vi "FPGAmain_5782_AM_PID_v2.vi"() -> ()   [LabVIEW 2013]
uses:
  FPGA/DataMode.ctl
  FPGA/Input_5782/5782_states.ctl
  <vilib>/Platform/TimedLoop/XDataNode/timing_clust.ctl
  <vilib>/Platform/TimedLoop/XDataNode/nitl_modes.ctl
  <vilib>/Platform/TimedLoop/XDataNode/wakeup.ctl
  <vilib>/rvi/Emulation/niFpgaSctlEmulationGetInTimedLoop.vi
  <vilib>/rvi/Emulation/niFpgaEmulationReportErrorSimple.vi
  <vilib>/rvi/Emulation/niFpgaGetClockAttributes.vi
  <vilib>/rvi/eio/common/nirviEmuTemplateMethod_errors.vi
  <vilib>/rvi/Emulation/niFpgaCriticalErrorInLSC.vi
  <vilib>/rvi/DataTransferAndStorage/Register/Emulation/niFpgaRegisterEmulationFpgaImpl.vi
  <instcachedir>/0/niFpgaRegisterEmulationFpgaImpl_DCF4BC0110594B98B44A971D60CEEC4D.lvgen/niFpgaRegisterEmulationFpgaImpl_DCF4BC0110594B98B44A971D60CEEC4D_005.vi
  <vilib>/rvi/DataTransferAndStorage/Container/Common/niFpgaContainerGetUniqueNameForEmu.vi
  <instcachedir>/0/niFpgaRegisterEmulationFpgaImpl_DCF4BC0110594B98B44A971D60CEEC4D.lvgen/niFpgaRegisterEmulationFpgaImpl_DCF4BC0110594B98B44A971D60CEEC4D_016.vi
  <instcachedir>/0/niFpgaRegisterEmulationFpgaImpl_DCF4BC0110594B98B44A971D60CEEC4D.lvgen/niFpgaRegisterEmulationFpgaImpl_DCF4BC0110594B98B44A971D60CEEC4D_017.vi
  <instcachedir>/0/niFpgaRegisterEmulationFpgaImpl_DCF4BC0110594B98B44A971D60CEEC4D.lvgen/niFpgaRegisterEmulationFpgaImpl_DCF4BC0110594B98B44A971D60CEEC4D_012.vi
  <instcachedir>/0/niFpgaRegisterEmulationFpgaImpl_DCF4BC0110594B98B44A971D60CEEC4D.lvgen/niFpgaRegisterEmulationFpgaImpl_DCF4BC0110594B98B44A971D60CEEC4D_015.vi
  <vilib>/rvi/FIFO/Fifo_Resource/nirvififoEmulationReadFpgaImpl.vi
  <vilib>/rvi/interface/RandomDataEmulation/nirviRandomDataMultiElementFPGAFIFO.vi
  <instcachedir>/0/nirviRandomDataMultiElementFPGAFIFO_F2B80EDE0D7944A08478D8D26097D4DB.lvgen/nirviRandomDataMultiElementFPGAFIFO_F2B80EDE0D7944A08478D8D26097D4DB_005.vi
  <vilib>/rvi/interface/RandomDataEmulation/niFpgaRandomDataHandleErrors.vi
  <instcachedir>/0/niFpgaRegisterEmulationFpgaImpl_DCF4BC0110594B98B44A971D60CEEC4D.lvgen/niFpgaRegisterEmulationFpgaImpl_DCF4BC0110594B98B44A971D60CEEC4D_009.vi
  <vilib>/rvi/interface/RandomDataEmulation/nirviRandomDataFPGAFIFO.vi
  <vilib>/rvi/FIFO/Fifo_Resource/nirvififoEmulationWriteFpgaImpl.vi
  <vilib>/Platform/TimedLoop/XDataNode/XDataNode.xnode
  <vilib>/eio/EIONode/EIONode.xnode
  <vilib>/rvi/DataTransferAndStorage/Container/XNode/niFpgaContainer.xnode
  <vilib>/rvi/DataTransferAndStorage/Register/Emulation/niFpgaRegisterEmulation.vi
  <vilib>/rvi/FIFO/Fifo_Resource/nirvififoEmulationRead.vi
  <vilib>/rvi/interface/RandomDataEmulation/nirviRandomDataFpgaMultiElementTemplate.vi
  <vilib>/rvi/interface/RandomDataEmulation/nirviRandomDataFpgaReadWriteTemplate.vi
  <vilib>/rvi/FIFO/Fifo_Resource/nirvififoEmulationWrite.vi
  <vilib>/Platform/TimedLoop/XDataNode/XDNodeRunTimeDep.lvlib
panel:
  in  "IO Module\\AO Data Sync":bool=TRUE
  in  "IO Module\\SPI Write Data":u16
  out "IO Module\\SPI Read Data":u8
  in  "IO Module\\SPI Read":bool
  in  "IO Module\\SPI Write":bool
  in  "IO Module\\SPI Address":u16
  in  "IO Module\\SPI Device":u8
  out "IO Module\\SPI Idle":bool
  in  "AM phase":fxp<+,64,64>
  in  "delay phase":fxp<+,64,64>
  in  "User Command Commit":bool
  in  "User Command":u8
  out "User Command Idle":bool
  out "User Command Status":u8
  in  "User Data 0":u8
  in  "User Data 1":u8
  out "PLL Locked":bool
  out "User Error":bool
  out "Configured?":bool
  in  "Continuous":bool
  in  "5782 record length":u16=4000 caption="Samples Per Trigger" min=1 step=1
  in  "Trigger Acquisition":bool
  out "IO Module\\Trigger Input":bool
  in  "Downsample":fxp<+,8,8>=1.0
  in  "new coeffs":bool
  in  "FIR coeffs":fxp<+/-,18,18>[](array[numeric])
  in  "CIC Gain":fxp<+/-,32,1>=0.00390625 format="%#_32g"
  in  "Acquisition running":bool
  in  "Phase output":fxp<+,64,64>[](array[numeric])=[0.0, 0.0, 0.0, 0.0, 0.0, 0.0, 0.0, 0.0]
  in  "Simulated phase 5782":fxp<+,64,64>[](array[numeric])=[0.0, 0.0]
  in  "Mode":T1
  in  "Phase 5782":fxp<+,64,64>[](array[numeric])=[0.0, 0.0]
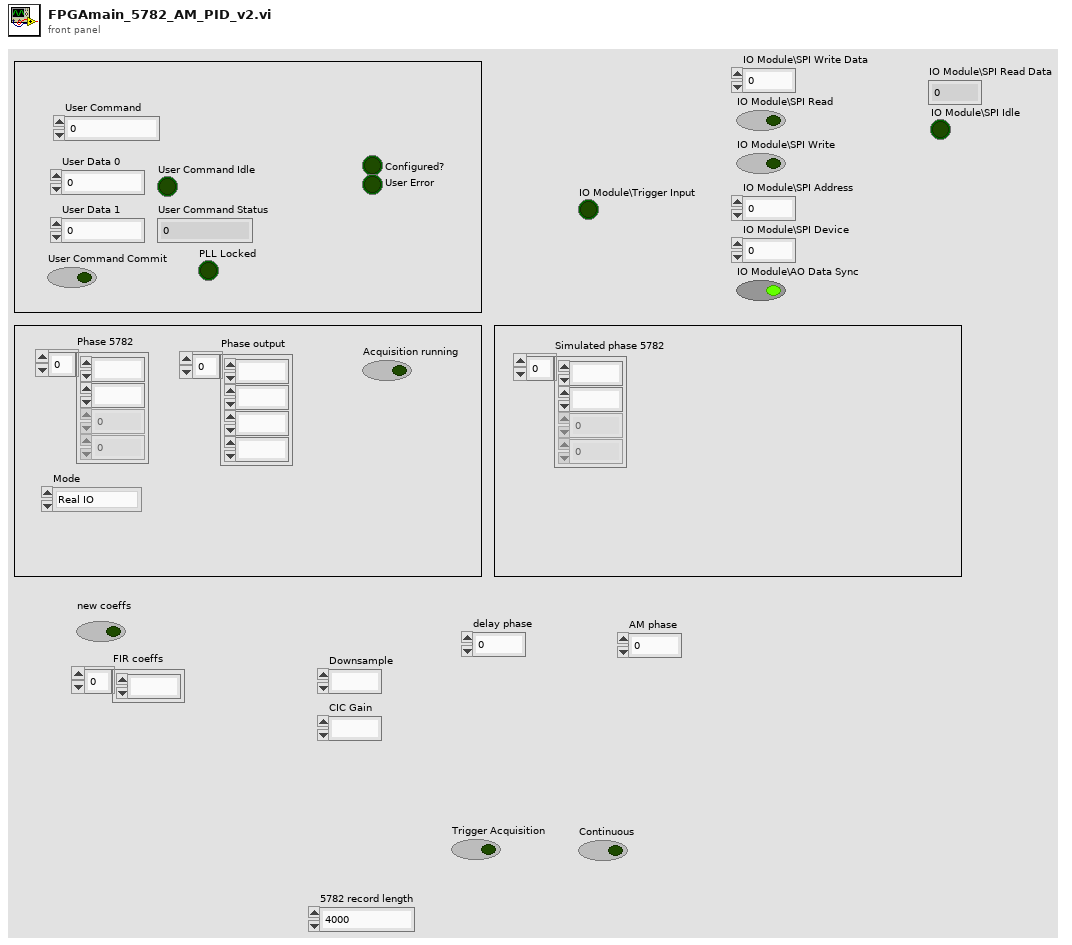
[diagram p1: front panel]
types:
  T1 = typedef "DataMode.ctl" = enum16{"Real IO", "Simulated"}
  T2 = typedef "5782_states.ctl" = enum8{"Wait for trigger", "Acquisition", "Send record length", "Quiet period"}
  T3 = typedef "XDNodeRunTimeDep.lvlib/timing_clust.ctl" = cluster{"Expected End [f-1]":u64, "Actual End [f-1]":u64, "Finished Late? [f-1]":bool, "Expected End [i-1]":u64, "Actual End [i-1]":u64, "Finished Late? [i-1]":bool, "Expected Start [i]":u64, "Actual Start [i]":u64, "Expected Start [f]":u64, "Actual Start [f]":u64, "Source Name":string, "Structure Name":string, "Period":i64, "Deadline":i64, "Offset":i64, "Start":i64, "Priority":i32, "Timeout":i32, "Mode":T4, "Wakeup Reason":T5, "Error":errorcluster, "Source Type":string, "Secondary Source Type":string, "Global End Time":u64, "Global Start Time":u64, "Frame Duration":u64, "Iteration Duration":u64, "Assigned CPU":i32, "I/O Scan Engine Mode":u32}
  T4 = typedef "XDNodeRunTimeDep.lvlib/nitl_modes.ctl" = enum32{"No Change", "Process missed periods, maintain original phase", "Discard missed periods, maintain original phase", "Process missed periods, ignore original phase", "Discard missed periods, ignore original phase"}
  T5 = typedef "XDNodeRunTimeDep.lvlib/wakeup.ctl" = enum32{"Normal", "Aborted", "Asynchronous wakeup", "Timing source error", "Timed loop error", "Timeout"}
  T6 = typedef "I16 array size 2.ctl" = i16[]
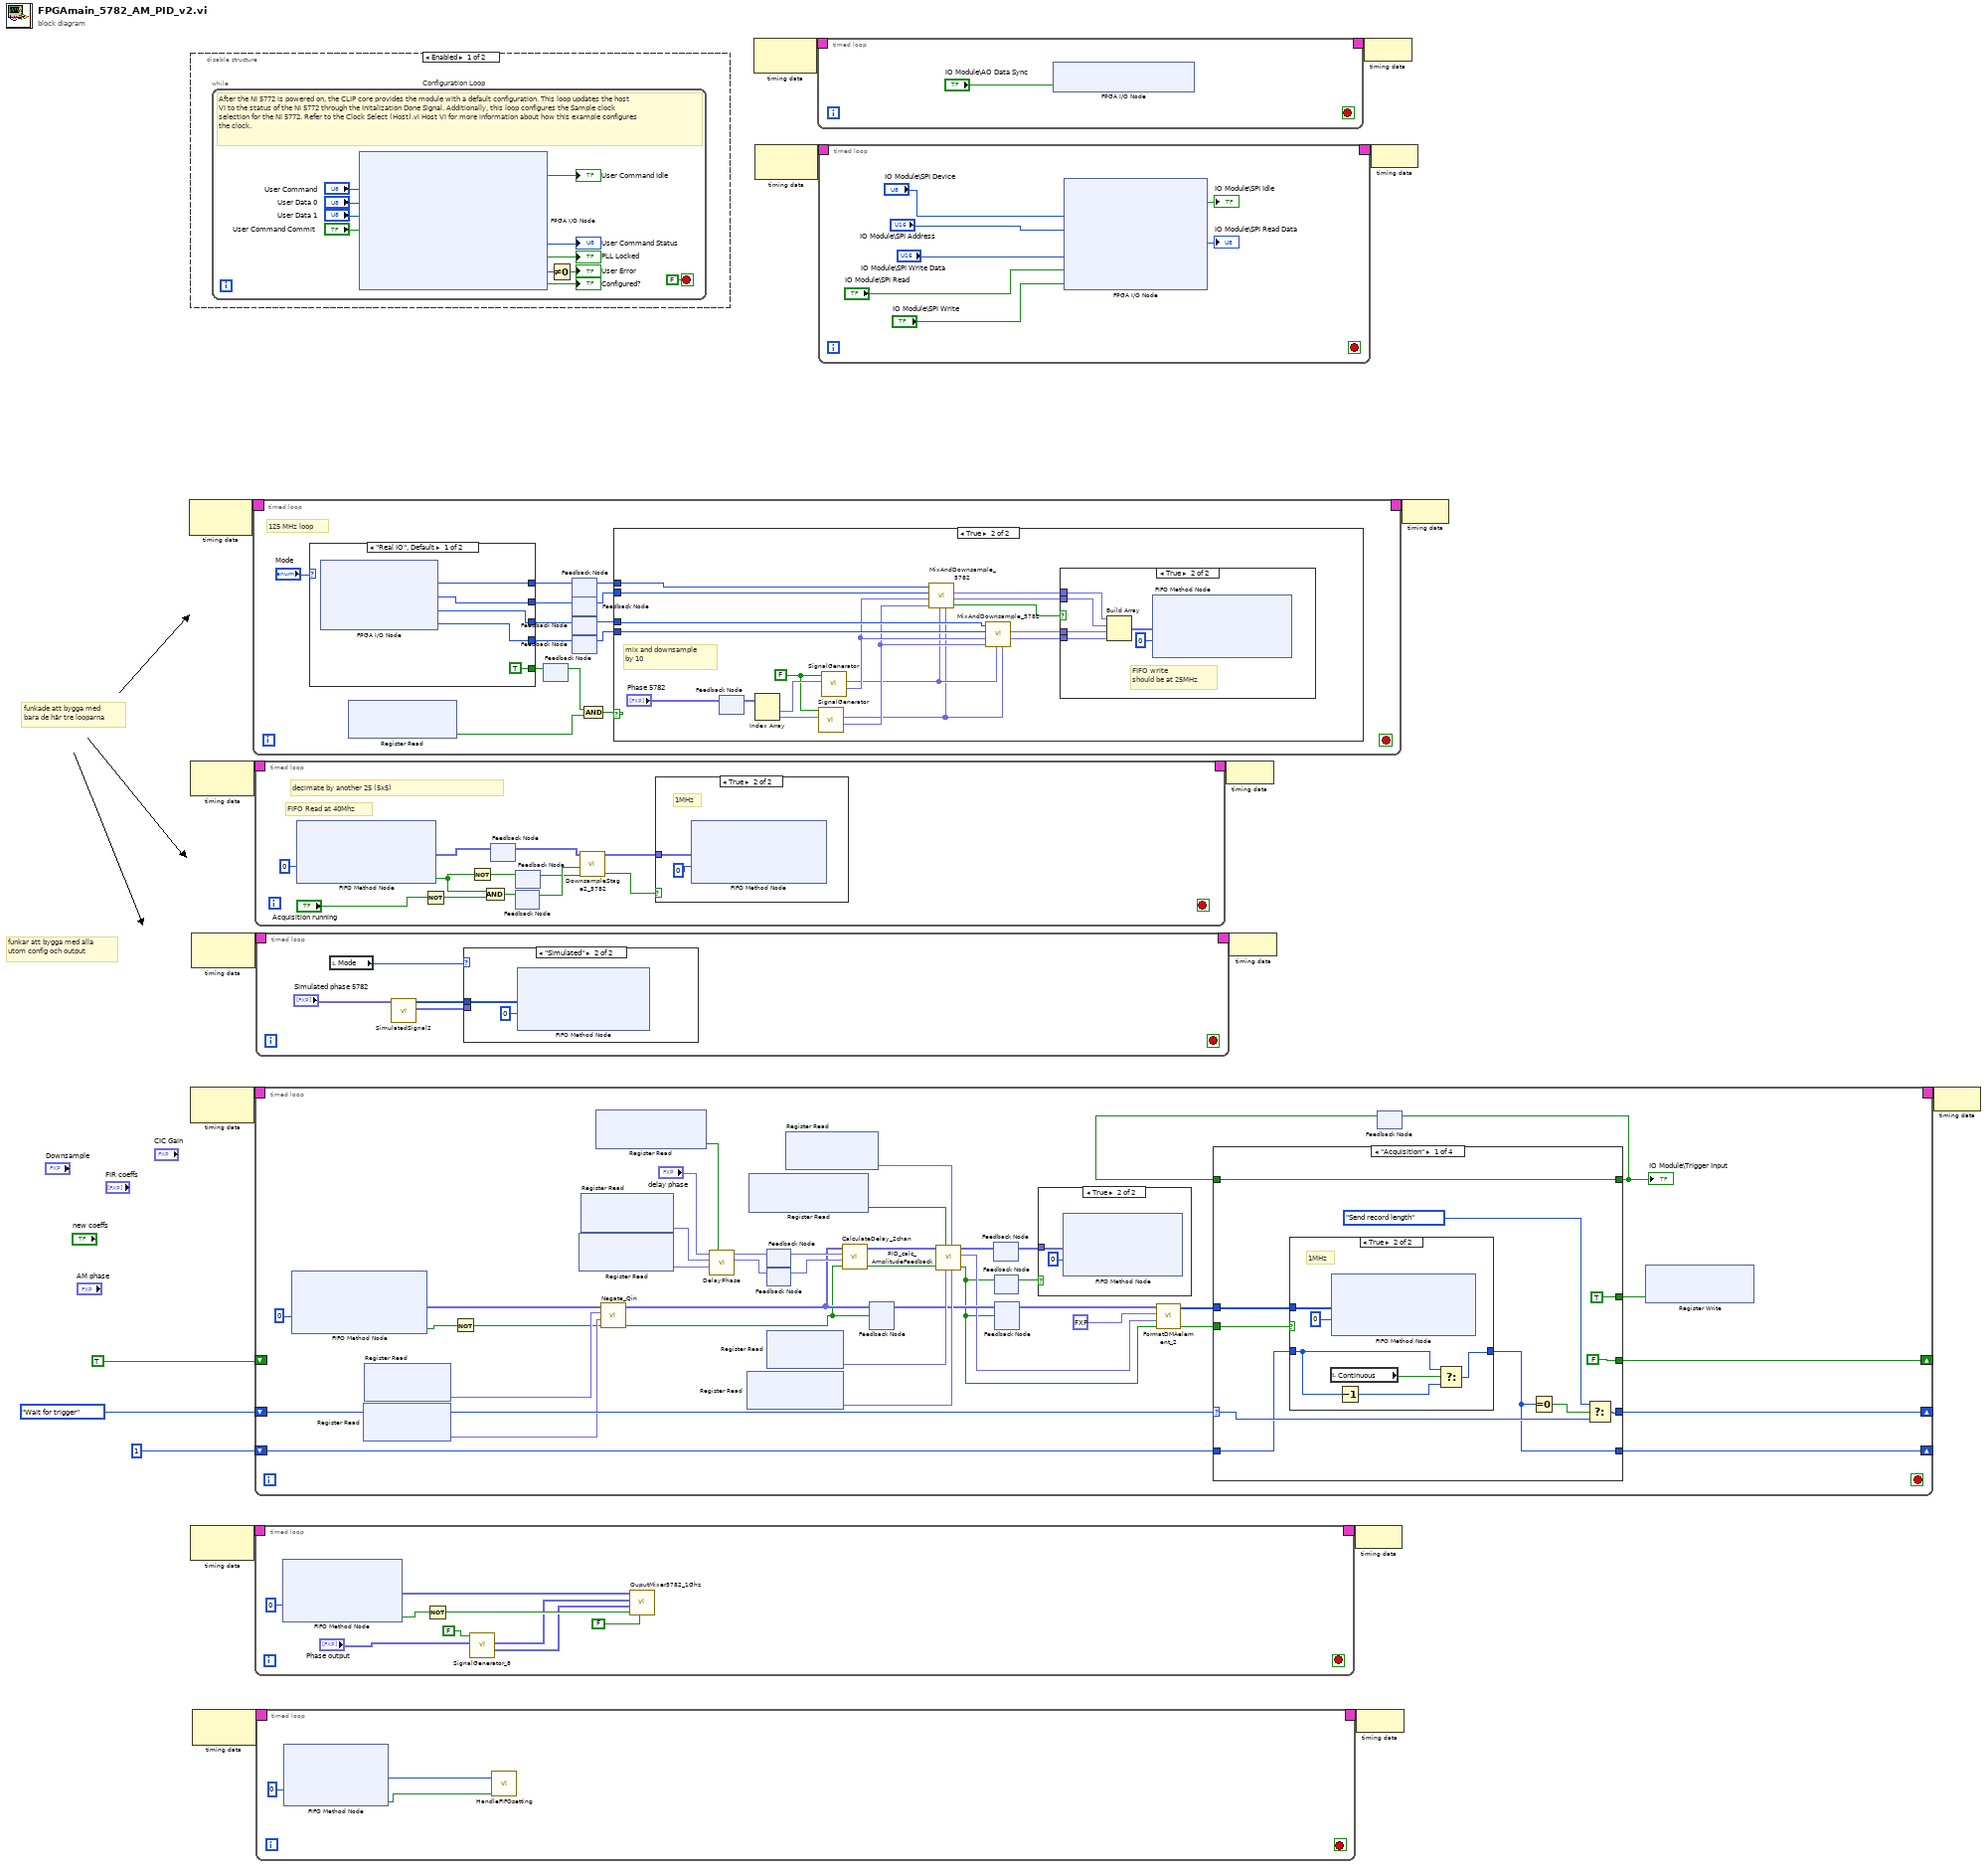
[diagram p0: block diagram]
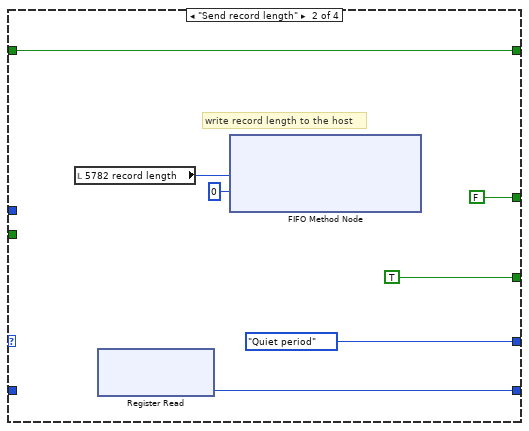
[diagram p4: hidden frame]
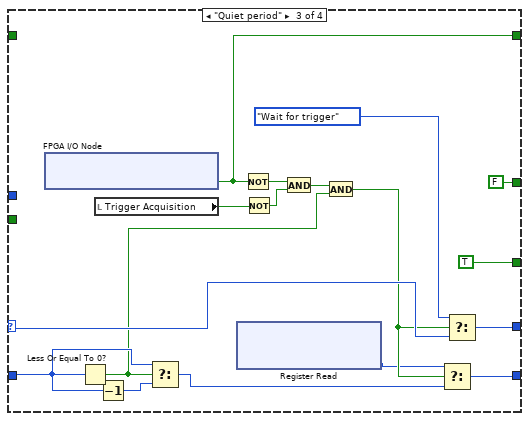
[diagram p5: hidden frame]
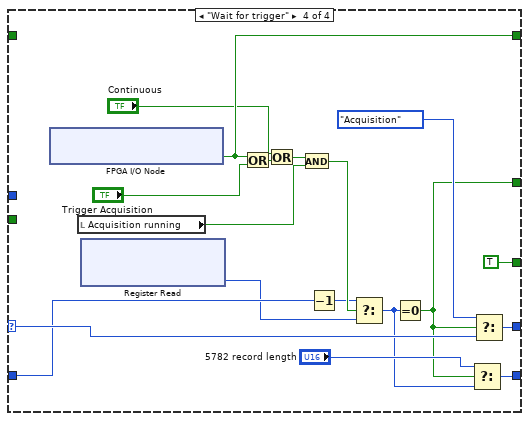
[diagram p6: hidden frame]
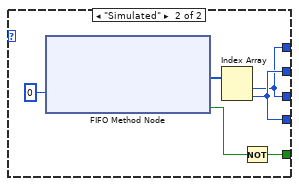
[diagram p10: hidden frame]
diagram:
  # "funkar att bygga med alla\nutom config och output"
  # "funkade att bygga med\nbara de här tre looparna"
  n1 = node-c288() -> (w15:T3)  [unwired: 1 in]
  n2 = disable-structure shown="Enabled" {
    frame Enabled {
      n3 = while "Configuration Loop" {
        stop <- FALSE stop-if-true
        # "After the NI 5772 is powered on, the CLIP core provides the module with a default configuration. This loop updates the host VI to the status of the NI 5772 through the Initalization Done Signal. Additionally, this loop configures the Sample clock selection for the NI 5772. Refer to the Clock Select (Host).vi Host VI for more information about how this example configures the clock."
        n4 = xnode "FPGA I/O Node"("IO Module\\User Command"="User Command", "IO Module\\User Data 0"="User Data 0", "IO Module\\User Data 1"="User Data 1", "IO Module\\User Command Commit"="User Command Commit") -> ("IO Module\\User Command Idle"=→"User Command Idle":bool, "IO Module\\User Command Status"=→"User Command Status":u8, "IO Module\\PLL Locked"=→"PLL Locked":bool, "IO Module\\User Error"=w25:u8, "IO Module\\Initialization Done"=→"Configured?":bool)  [unwired: 9 in, 9 out]
        n5 = Not Equal To 0?(x=w25) -> (x != 0?=→"User Error":bool)
      }
    }
    frame Disabled {
    }
  }
  n6 = node-c288() -> (w19:T3)  [unwired: 1 in]
  n7 = node-c288() -> (w13:T3)  [unwired: 1 in]
  n8 = node-c288() -> (w6:T3)  [unwired: 1 in]
  n9 = node-c288() -> (w17:T3)  [unwired: 1 in]
  n10 = node-c288() -> (w8:T3)  [unwired: 1 in]
  n11 = timed-loop {
    timing: w15 -> [_]
    timing-out: [_] -> w14
    stop <- _ stop-if-true
    # "125 MHz loop"
    n12 = case shown="\"Real IO\", Default" "Mode" {
      tunnel: [w72 w75] -> w41
      tunnel: [w71 w76] -> w39
      tunnel: [w70 w75] -> w37
      tunnel: [w69 w76] -> w34
      tunnel: [TRUE w73] -> w33
      frame "Real IO", Default {
        n13 = xnode "FPGA I/O Node"() -> ("IO Module\\AI 0 N-1"=w72:i16, "IO Module\\AI 0 N"=w71:i16, "IO Module\\AI 1 N-1"=w70:i16, "IO Module\\AI 1 N"=w69:i16)  [unwired: 4 in, 4 out]
      }
      frame "Simulated" {
        n14 = xnode ("FIFO Method Node")("Timeout"=0) -> ("Element"=w77:i16[], "Timed Out?"=w74:bool)  [unwired: 1 in, 1 out]
        n15 = Index Array(array=w77) -> (element #1=w75:i16, element #2=w76:i16)  [unwired: 2 in]
        n16 = Not(x=w74) -> (.not. x?=w73:bool)
      }
    }
    n17 = xnode ("Register Read")() -> ("Data"=w31:bool)  [unwired: 1 in, 1 out]
    n18 = feedback #1() -> (w32:bool)  [unwired: 1 in]
    n19 = feedback-in #1(w33) -> ()
    n20 = feedback #2() -> (w40:i16)  [unwired: 1 in]
    n21 = feedback-in #2(w41) -> ()
    n22 = feedback #3() -> (w38:i16)  [unwired: 1 in]
    n23 = feedback-in #3(w39) -> ()
    n24 = feedback #4() -> (w36:i16)  [unwired: 1 in]
    n25 = feedback-in #4(w37) -> ()
    n26 = feedback #5() -> (w35:i16)  [unwired: 1 in]
    n27 = feedback-in #5(w34) -> ()
    n28 = And(x=w32, y=w31) -> (x .and. y?=w42:bool)
    n29 = case shown="True" w42 {
      tunnel: w40 -> [_ w51]
      tunnel: w38 -> [_ w50]
      tunnel: w36 -> [_ w49]
      tunnel: w35 -> [_ w48]
      frame False {
      }
      frame True {
        w52 = FALSE
        # "mix and downsample\nby 10"
        n30 = feedback #6() -> (w55:fxp<+,64,64>[])  [unwired: 1 in]
        n31 = feedback-in #6("Phase 5782") -> ()
        n32 = Index Array(array=w55) -> (element #1=w54:fxp<+,64,64>, element #2=w56:fxp<+,64,64>)  [unwired: 2 in]
        n33 = call "SignalGenerator.vi"("phase"=w56, "Reset"=w52) -> ("Cos"=w46:fxp<+/-,16,0>, "Sin"=w44:fxp<+/-,16,0>)  [unwired: 7 in, 1 out]
        n34 = call "SignalGenerator.vi"("phase"=w54, "Reset"=w52) -> ("Cos"=w47:fxp<+/-,16,0>, "Sin"=w45:fxp<+/-,16,0>)  [unwired: 7 in, 1 out]
        n35 = call "MixAndDownsample_5782.vi"("sin1"=w44, "sin0"=w45, "cos1"=w46, "cos0"=w47, "signal 1"=w50, "signal 0"=w51) -> ("data valid"=w59:bool, "Q out"=w60:fxp<+/-,16,14>, "I out"=w61:fxp<+/-,16,14>)  [unwired: 3 in]
        n36 = call "MixAndDownsample_5782.vi"("sin1"=w44, "sin0"=w45, "cos1"=w46, "cos0"=w47, "signal 1"=w48, "signal 0"=w49) -> ("Q out"=w57:fxp<+/-,16,14>, "I out"=w58:fxp<+/-,16,14>)  [unwired: 3 in, 1 out]
        n37 = case shown="True" w59 {
          tunnel: w60 -> [_ w67]
          tunnel: w61 -> [_ w64]
          tunnel: w58 -> [_ w63]
          tunnel: w57 -> [_ w62]
          frame False {
          }
          frame True {
            # "FIFO write\nshould be at 25MHz"
            n38 = Build Array(w64, w67, w63, w62) -> (w66:fxp<+/-,16,14>[])
            n39 = xnode ("FIFO Method Node")("Element"=w66, "Timeout"=0) -> ()  [unwired: 1 in, 2 out]
          }
        }
      }
    }
  }
  n40 = timed-loop {
    timing: w19 -> [_]
    timing-out: [_] -> w18
    stop <- _ stop-if-true
    # "FIFO Read at 40Mhz"
    # "decimate by another 25 (5x5)"
    n41 = xnode ("FIFO Method Node")("Timeout"=0) -> ("Element"=w86:fxp<+/-,16,14>[], "Timed Out?"=w88:bool)  [unwired: 1 in, 1 out]
    n42 = Not(x="Acquisition running") -> (.not. x?=w89:bool)
    n43 = Not(x=w88) -> (.not. x?=w82:bool)
    n44 = And(x=w88, y=w89) -> (x .and. y?=w84:bool)
    n45 = feedback #7() -> (w85:fxp<+/-,16,14>[])  [unwired: 1 in]
    n46 = feedback-in #7(w86) -> ()
    n47 = feedback #8() -> (w83:bool)  [unwired: 1 in]
    n48 = feedback-in #8(w84) -> ()
    n49 = feedback #9() -> (w81:bool)  [unwired: 1 in]
    n50 = feedback-in #9(w82) -> ()
    n51 = call "DownsampleStage2_5782.vi"("valid in"=w81, "reset"=w83, "Data in"=w85) -> ("valid out"=w90:bool, "data out"=w91:fxp<+/-,16,14>[])  [unwired: 7 in]
    n52 = case shown="True" w90 {
      tunnel: w91 -> [_ w93]
      frame False {
      }
      frame True {
        # "1MHz"
        n53 = xnode ("FIFO Method Node")("Element"=w93, "Timeout"=0) -> ()  [unwired: 1 in, 2 out]
      }
    }
  }
  n54 = timed-loop {
    timing: w13 -> [_]
    timing-out: [_] -> w12
    shift-right: [w134] -> _
    shift-left: 5782_states."Wait for trigger" ("5782 states") -> [w136]
    shift-right: [w133] -> _
    shift-left: u16 1 ("trigger samples") -> [w135]
    shift-right: [w128] -> _
    shift-left: TRUE -> [_]
    stop <- _ stop-if-true
    n55 = xnode ("FIFO Method Node")("Timeout"=0) -> ("Element"=w107:fxp<+/-,16,14>[], "Timed Out?"=w131:bool)  [unwired: 1 in, 1 out]
    n56 = xnode ("Register Read")() -> ("Data"=w118:fxp<+/-,16,14>)  [unwired: 1 in, 1 out]
    n57 = xnode ("Register Read")() -> ("Data"=w119:fxp<+/-,16,14>)  [unwired: 1 in, 1 out]
    n58 = Not(x=w131) -> (.not. x?=w108:bool)
    n59 = xnode ("Register Read")() -> ("Data"=w115:fxp<+/-,16,0>)  [unwired: 1 in, 1 out]
    n60 = xnode ("Register Read")() -> ("Data"=w116:fxp<+/-,16,0>)  [unwired: 1 in, 1 out]
    n61 = xnode ("Register Read")() -> ("Data"=w117:bool)  [unwired: 1 in, 1 out]
    n62 = call "Negate_Qin.vi"("valid in"=w108, "DC offset chan 1"=w118, "DC offset chan 0"=w119, "Data in"=w107) -> ("valid out"=w101:bool, "Data out"=w102:fxp<+/-,16,14>[])  [unwired: 6 in]
    n63 = call "DelayPhase.vi"("Use fixed delay"=w117, "fixed cos_fi"=w115, "fixed sin fi"=w116, "delay phase"="delay phase") -> ("cos_fi"=w120:fxp<+/-,16,0>, "sin fi"=w121:fxp<+/-,16,0>)  [unwired: 6 in]
    n64 = xnode ("Register Read")() -> ("Data"=w110:fxp<+/-,32,6>)  [unwired: 1 in, 1 out]
    n65 = xnode ("Register Read")() -> ("Data"=w112:bool)  [unwired: 1 in, 1 out]
    n66 = feedback-in #10(w121) -> ()
    n67 = feedback #10() -> (w124:fxp<+/-,16,0>)  [unwired: 1 in]
    n68 = feedback #11() -> (w123:fxp<+/-,16,0>)  [unwired: 1 in]
    n69 = feedback-in #11(w120) -> ()
    n70 = xnode ("Register Read")() -> ("Data"=w111:fxp<+/-,32,6>)  [unwired: 1 in, 1 out]
    n71 = xnode ("Register Read")() -> ("Data"=w109:fxp<+/-,32,6>)  [unwired: 1 in, 1 out]
    n72 = call "CalculateDelay_2chan.vi"("input valid"=w101, "cos_fi"=w123, "sin fi"=w124, "Data in"=w102) -> ("output valid"=w113:bool, "Data out"=w114:fxp<+/-,16,14>[])  [unwired: 6 in]
    n73 = feedback #12() -> (w103:fxp<+/-,16,14>[])  [unwired: 1 in]
    n74 = feedback-in #12(w102, w101) -> ()
    n75 = call "PID_calc_AmplitudeFeedback.vi"("Kd/Tau"=w110, "Ki*Tau"=w109, "Kp"=w111, "Enabled"=w112, "input valid"=w113, "Data in"=w114) -> ("output valid"=w97:bool, "c(t)"=w99:fxp<+/-,32,21>, "data out"=w106:fxp<+/-,16,14>[])  [unwired: 2 in, 1 out]
    n76 = feedback #13() -> (w105:fxp<+/-,16,14>[])  [unwired: 1 in]
    n77 = feedback-in #13(w106) -> ()
    n78 = feedback #14() -> (w104:bool)  [unwired: 1 in]
    n79 = feedback-in #14(w97) -> ()
    n80 = feedback #15() -> (w100:fxp<+/-,16,14>[])  [unwired: 1 in]
    n81 = feedback-in #15(w103, w97) -> ()
    n82 = case shown="True" w104 {
      tunnel: w105 -> [_ w137]
      frame False {
      }
      frame True {
        n83 = xnode ("FIFO Method Node")("Element"=w137, "Timeout"=0) -> ()  [unwired: 1 in, 2 out]
      }
    }
    n84 = call "FormatDMAelement_2.vi"("valid in"=w97, "c(t) - AM"=w99, "c(t) - Phase"=fxp<+/-,32,21> 0.0, "Data in"=w100) -> ("valid out"=w129:bool, "Element"=w130:u64[])  [unwired: 6 in]
    n85 = feedback #16() -> (w126:bool)  [unwired: 1 in]
    n86 = case shown="\"Acquisition\"" w136 {
      selector: w136 -> [w149 _ w179 w198]
      tunnel: w135 -> [w145 _ w167 w185]
      tunnel: [w148 5782_states."Quiet period" ("5782 states") w178 w197] -> w134
      tunnel: [w142 w157 w180 w196] -> w133
      tunnel: w130 -> [w143 _ _ _]
      tunnel: w129 -> [w144 _ _ _]
      tunnel: [FALSE TRUE TRUE TRUE] -> w128
      tunnel: [TRUE FALSE ("5782 triggered") FALSE ("5782 triggered") w189] -> w127
      tunnel: [w141 w158 w169 w188] -> w125
      tunnel: w126 -> [w141 w158 _ _]
      frame "Acquisition" {
        n87 = case shown="True" w144 {
          tunnel: w143 -> [_ w156]
          tunnel: [w150 w153] -> w142
          tunnel: w145 -> [w150 w151]
          frame False {
          }
          frame True {
            # "1MHz"
            n88 = local read "Continuous"() -> (w154:bool)
            n89 = xnode ("FIFO Method Node")("Element"=w156, "Timeout"=0) -> ()  [unwired: 1 in, 2 out]
            n90 = Decrement(x=w151) -> (x-1=w152:u16)
            n91 = Select(t=w151, s=w154, f=w152) -> (s? t:f=w153:u16)
          }
        }
        n92 = Equal To 0?(x=w142) -> (x = 0?=w146:bool)
        n93 = Select(t=5782_states."Send record length" ("5782 states"), s=w146, f=w149) -> (s? t:f=w148:T2)
      }
      frame "Send record length" {
        # "write record length to the host"
        n94 = local read "5782 record length"() -> (w160:u16)
        n95 = xnode ("Register Read")() -> ("Data"=w157:u16)  [unwired: 1 in, 1 out]
        n96 = xnode ("FIFO Method Node")("Element"=w160, "Timeout"=0) -> ()  [unwired: 1 in, 2 out]
      }
      frame "Quiet period" {
        n97 = xnode "FPGA I/O Node"() -> ("IO Module\\Trigger Input"=w169:bool)  [unwired: 1 in, 1 out]
        n98 = Less Or Equal To 0?(x=w167) -> (x <= 0?=w166:bool)
        n99 = local read "Trigger Acquisition"() -> (w175:bool)
        n100 = Decrement(x=w167) -> (x-1=w168:u16)
        n101 = Select(t=w167, s=w166, f=w168) -> (s? t:f=w165:u16)
        n102 = xnode ("Register Read")() -> ("Data"=w164:u16)  [unwired: 1 in, 1 out]
        n103 = Not(x=w169) -> (.not. x?=w174:bool)
        n104 = Not(x=w175) -> (.not. x?=w173:bool)
        n105 = And(x=w174, y=w173) -> (x .and. y?=w172:bool)
        n106 = And(x=w172, y=w166) -> (x .and. y?=w177:bool)
        n107 = Select(t=w164, s=w177, f=w165) -> (s? t:f=w180:u16)
        n108 = Select(t=5782_states."Wait for trigger" ("5782 states"), s=w177, f=w179) -> (s? t:f=w178:T2)
      }
      frame "Wait for trigger" {
        n109 = xnode "FPGA I/O Node"() -> ("IO Module\\Trigger Input"=w188:bool)  [unwired: 1 in, 1 out]
        n110 = local read "Acquisition running"() -> (w190:bool)
        n111 = xnode ("Register Read")() -> ("Data"=w181:u16)  [unwired: 1 in, 1 out]
        n112 = Or(x=w188, y="Trigger Acquisition") -> (x .or. y?=w184:bool)
        n113 = Or(x="Continuous", y=w184) -> (x .or. y?=w182:bool)
        n114 = And(x=w182, y=w190) -> (x .and. y?=w191:bool)
        n115 = Decrement(x=w185) -> (x-1=w186:u16)
        n116 = Select(t=w186, s=w191, f=w181) -> (s? t:f=w187:u16)
        n117 = Equal To 0?(x=w187) -> (x = 0?=w189:bool)
        n118 = Select(t="5782 record length", s=w189, f=w187) -> (s? t:f=w196:u16)
        n119 = Select(t=5782_states."Acquisition" ("5782 states"), s=w189, f=w198) -> (s? t:f=w197:T2)
      }
    }
    "IO Module\\Trigger Input" <- w125
    n120 = feedback-in #16(w125) -> ()
    n121 = xnode ("Register Write")("Data"=w127) -> ()  [unwired: 1 in, 1 out]
  }
  n122 = timed-loop {
    timing: w6 -> [_]
    timing-out: [_] -> w5
    stop <- _ stop-if-true
    n123 = xnode ("FIFO Method Node")("Timeout"=0) -> ("Element"=w205:fxp<+/-,16,14>[], "Timed Out?"=w208:bool)  [unwired: 1 in, 1 out]
    n124 = Not(x=w208) -> (.not. x?=w204:bool)
    n125 = call "SignalGenerator_8.vi"("Phase"="Phase output", "reset"=FALSE) -> ("Sine out"=w201:fxp<+/-,16,0>[], "Cosine out"=w202:fxp<+/-,16,0>[])  [unwired: 8 in]
    n126 = call "OuputMixer5782_1Ghz.vi"("reset"=FALSE, "valid in"=w204, "Sine in"=w201, "Cosine in"=w202, "Data in"=w205) -> ()  [unwired: 5 in, 2 out]
  }
  n127 = timed-loop {
    timing: w17 -> [_]
    timing-out: [_] -> w16
    stop <- _ stop-if-true
    n128 = local read "Mode"() -> (w215:T1)
    n129 = call "SimulatedSignal2.vi"("Phase"="Simulated phase 5782") -> ("dummy do not use"=w212:fxp<+/-,16,0>[], "output"=w214:T6)  [unwired: 9 in]
    n130 = case shown="\"Simulated\"" w215 {
      tunnel: w214 -> [_ w216]
      tunnel: w212 -> [_ _]
      frame "Real IO", Default {
      }
      frame "Simulated" {
        n131 = xnode ("FIFO Method Node")("Element"=w216, "Timeout"=0) -> ()  [unwired: 1 in, 2 out]
      }
    }
  }
  n132 = timed-loop {
    timing: w8 -> [_]
    timing-out: [_] -> w7
    stop <- _ stop-if-true
    n133 = xnode ("FIFO Method Node")("Timeout"=0) -> ("Element"=w221:u64, "Timed Out?"=w220:bool)  [unwired: 1 in, 1 out]
    n134 = call "HandleFIFOsetting.vi"("timed out"=w220, "Value"=w221) -> ()  [unwired: 10 in]
  }
  n135 = node-c288() -> (w2:T3)  [unwired: 1 in]
  n136 = node-c288() -> (w4:T3)  [unwired: 1 in]
  n137 = timed-loop {
    timing: w2 -> [_]
    timing-out: [_] -> w1
    stop <- _ stop-if-true
    n138 = xnode "FPGA I/O Node"("IO Module\\AO Data Sync"="IO Module\\AO Data Sync") -> ()  [unwired: 1 in, 1 out]
  }
  n139 = timed-loop {
    timing: w4 -> [_]
    timing-out: [_] -> w3
    stop <- _ stop-if-true
    n140 = xnode "FPGA I/O Node"("IO Module\\SPI Device"="IO Module\\SPI Device", "IO Module\\SPI Address"="IO Module\\SPI Address", "IO Module\\SPI Write Data"="IO Module\\SPI Write Data", "IO Module\\SPI Read"="IO Module\\SPI Read", "IO Module\\SPI Write"="IO Module\\SPI Write") -> ("IO Module\\SPI Idle"=→"IO Module\\SPI Idle":bool, "IO Module\\SPI Read Data"=→"IO Module\\SPI Read Data":u8)  [unwired: 7 in, 7 out]
  }
  n141 = node-c288(w18) -> ()
  n142 = node-c288(w16) -> ()
  n143 = node-c288(w5) -> ()
  n144 = node-c288(w7) -> ()
  n145 = node-c288(w1) -> ()
  n146 = node-c288(w3) -> ()
  n147 = node-c288(w14) -> ()
  n148 = node-c288(w12) -> ()
